vi "EnFlo_Hub.vi"() -> ()   [LabVIEW 2010]
uses:
  Anemometry Sub Vis/Controls/Launch_controls/Open_Calib.ctl
  Anemometry Sub Vis/Controls/Launch_controls/Open_Meas.ctl
  Anemometry Sub Vis/Controls/Launch_controls/Open_Enter_Temp.ctl
  Anemometry Sub Vis/Controls/Launch_controls/Multi_Run_Prog.ctl
  Anemometry Sub Vis/Controls/Launch_controls/EnFlo_arm.ctl
  Anemometry Sub Vis/Controls/Launch_controls/Fast_FID_Valve.ctl
  Anemometry Sub Vis/Controls/Launch_controls/Disp_Setup.ctl
  Anemometry Sub Vis/Controls/Launch_controls/EnFlo_Tun_Setup.ctl
  Anemometry Sub Vis/Controls/Launch_controls/User_Metadata.ctl
  Anemometry Sub Vis/Controls/Launch_controls/Trav_3D_move.ctl
  Anemometry Sub Vis/Controls/Launch_controls/Trav_Space.ctl
  Anemometry Sub Vis/Controls/Launch_controls/Tunnel_speed.ctl
  Anemometry Sub Vis/Controls/Launch_controls/Client_source_control.ctl
  Anemometry Sub Vis/Controls/Launch_controls/Hydrosonic_Manual.ctl
  Anemometry Sub Vis/Controls/Launch_controls/Preference_Panel.ctl
  Anemometry Sub Vis/Controls/Launch_controls/Hot_wire_Calculator.ctl
  Anemometry Sub Vis/Controls/Launch_controls/RW_X_Parker_Config.ctl
  Anemometry Sub Vis/Controls/Launch_controls/LDA_Alignment.ctl
  Anemometry Sub Vis/Controls/Launch_controls/Named_Serial_Comms.ctl
  Anemometry Sub Vis/Controls/Launch_controls/BSA_data_rates.ctl
  Anemometry Sub Vis/Controls/Launch_controls/Recompile_Code.ctl
  Anemometry Sub Vis/Controls/Launch_controls/Serial_Setup.ctl
  Anemometry Sub Vis/Controls/Launch_controls/Post_Process_icon.ctl
  Anemometry Sub Vis/Controls/Launch_controls/Edit_Ascii_file.ctl
  Anemometry Sub Vis/Controls/Launch_controls/Edit_Raw_DF.ctl
  Anemometry Sub Vis/Controls/Launch_controls/Results_file_plotter.ctl
  Anemometry Sub Vis/Controls/Launch_controls/Serial_Port_Names.ctl
  Anemometry Sub Vis/Controls/Launch_controls/Enter_LDA_Setup.ctl
  Anemometry Sub Vis/Controls/Launch_controls/Paul.ctl
  Anemometry Sub Vis/Controls/Launch_controls/Tom.ctl
  Anemometry Sub Vis/Controls/Launch_controls/Scani_Valve.ctl
  Anemometry Sub Vis/Controls/Launch_controls/Edit_sever_Channel.ctl
  Anemometry Sub Vis/Controls/Launch_controls/Day_file_plotter.ctl
  Anemometry Sub Vis/Controls/Launch_controls/Plot_Sever_Data.ctl
  Anemometry Sub Vis/Controls/Launch_controls/Adam_Table.ctl
  Anemometry Sub Vis/Controls/Launch_controls/Active_Channel_Control.ctl
  Anemometry Sub Vis/Controls/Post_Process.ctl
  Anemometry Sub Vis/Controls/Setup.ctl
  Anemometry Sub Vis/Controls/Preference_Mode.ctl
  Anemometry Sub Vis/Controls/User_Specific_mode.ctl
  Anemometry Sub Vis/Gen Trav/Trav_mode.ctl
  Anemometry Sub Vis/File/Setup_Filetype.ctl
  Anemometry Sub Vis/Calibration/Calib_mode.ctl
  Anemometry Sub Vis/Controls/App_Global.ctl
  Anemometry Sub Vis/Globals/Dynamic_call_global.ph.vi
  Anemometry Sub Vis/Globals/Preference_global.vi
  Anemometry Sub Vis/Globals/Constants_global.vi
  Anemometry Sub Vis/Globals/Meas_global.vi
  <vilib>/Platform/browser.llb/Open URL in Default Browser (string).vi
  Anemometry Sub Vis/Globals/Trav_pos_global.vi
  Anemometry Sub Vis/Acquisition/PWA/PWAtasksGLOBAL.vi
  Anemometry Sub Vis/Globals/Qnet_Globals.vi
  Anemometry Sub Vis/Utilities/Email_transfer_global.vi
panel:
  out "List of ADAM channels to view":string[](array[string])
  out "List of ADAM control channels":string[](array[string])
  out "Analogue Dev Name":string="Dev2"
  out "Numeric":i32
  out "Rig Name":string="EnFlo Tunnel"
  out "All Users":path=path "/System Folder/Preferences/LabVIEW (EnFlo specific)/Meas Setups"
  out "Dummy Measurement":bool
  out "Ready to take data?":T1
  out "Local Site Root":path=path "/Lacie_20/paulhayden/Qnet/qnet"
  in  "stop":bool
  in  "Tab Control":T2(tab)
  in  "Tunnel Speed Control":T3
  in  "Traverse Space":T4
  in  "Trav 3D Move":T5 caption="3D Traverse Move"
  in  "User Metadata":T6
  in  "Multi Run Prog":T7
  in  "Enter Temp_Press":T8
  in  "Measurement Prog":T9 caption="Measurement"
  in  "Calibration Prog":T10 caption="Calibration"
  in  "Scani Valve":T11
  in  "LDA Alignment":T12
  in  "Hydrosonic Control":T13
  in  "Fast FID Valve":T14
  in  "Source Control":T15
  in  "Gas Release Setup":T16
  in  "EnFlo Tunnel Setup":T17
  in  "Heater Setup":bool caption="Inlet heater File"
  in  "EnFlo Arm":T18
  in  "Rig_Control":cluster{"Ch Name":string, "Boolean":bool}[](array[cluster])
  in  "ADAM Channels Control":T19 caption="Change Active Channels"
  in  "ADAM Scan Table":T20 caption="Run ADAM Scan Table"
  in  "Edit Server Channel":T21
  in  "Plot Server Channels":T22 caption="Plot Server Data"
  in  "Day Files Plotter":T23 caption="Plot Data From File"
  out "Current Values":cluster{"Ch Name":string, "Numeric":dbl}[](array[cluster])
  in  "Results File Plotter":T24
  in  "Edit Raw Data Files":T25
  in  "Edit ASCII File":T26
  in  "Post Process Raw Data":T27
  in  "LDA Setup":T28
  in  "Port Names":T29
  in  "Serial Setup":T30
  in  "Software Update":T31
  in  "LDA Data Rate":T32
  in  "Named Serial Comms":T33
  in  "RW Trav Setup":T34
  in  "Hot Wire Calc":T35
  in  "Preference Panel":T36
  in  "Tom Lawton t.lawton@surrey.ac.uk":T37 caption="For hardware support"
  in  "Paul Hayden p.hayden@surrey.ac.uk":T38 caption="For software support"
  in  "Online Manual":bool
  out "VI Name":string
  out "Iterations":i32
  # "Or give us a call on Tel: 01483 689545"
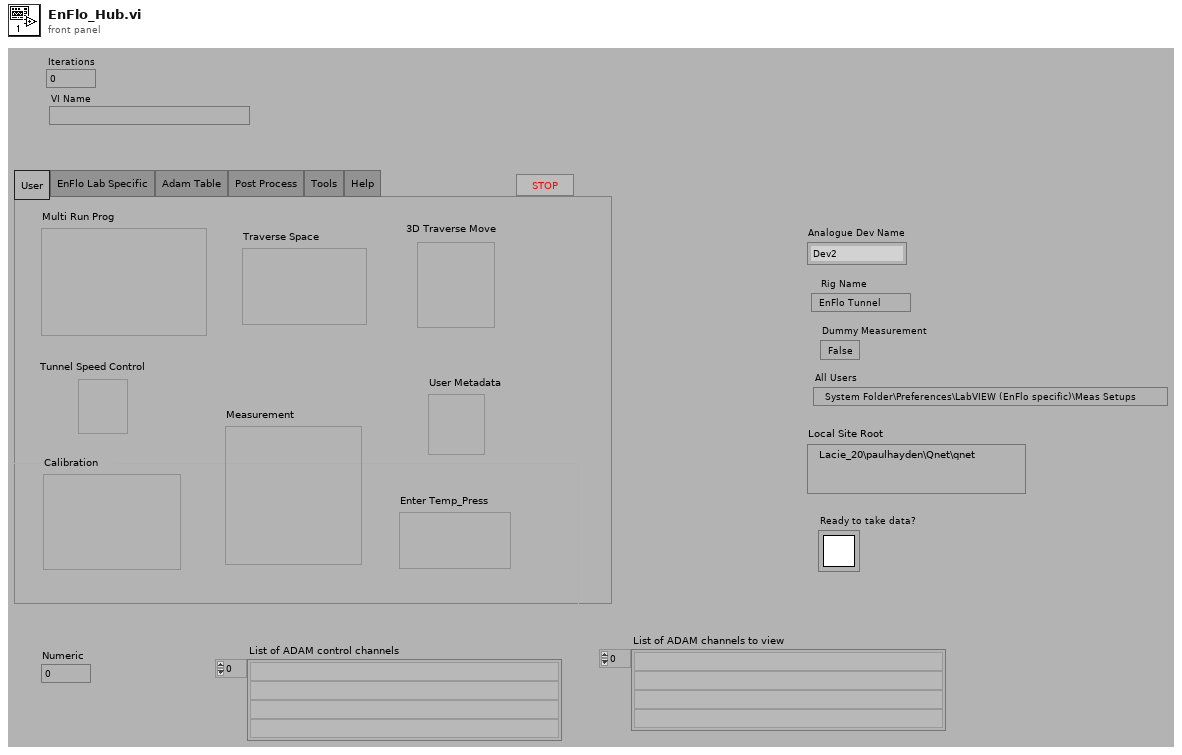
[diagram p1: front panel]
types:
  T1 = typedef "Rendezvous RefNum" = refnum<k1>
  T2 = enum32{"User", "EnFlo Lab Specific", "Adam Table", "Post Process", "Tools", "Help"}
  T3 = typedef "Tunnel_speed.ctl" = bool
  T4 = typedef "Trav_Space.ctl" = bool
  T5 = typedef "Trav_3D_move.ctl" = bool
  T6 = typedef "User_Metadata.ctl" = bool
  T7 = typedef "Multi_Run_Prog.ctl" = bool
  T8 = typedef "Open_Enter_Temp.ctl" = bool
  T9 = typedef "Open_Meas.ctl" = bool
  T10 = typedef "Open_Calib.ctl" = bool
  T11 = typedef "Scani_Valve.ctl" = bool
  T12 = typedef "LDA_Alignment.ctl" = bool
  T13 = typedef "Hydrosonic_Manual.ctl" = bool
  T14 = typedef "Fast_FID_Valve.ctl" = bool
  T15 = typedef "Client_source_control.ctl" = bool
  T16 = typedef "Disp_Setup.ctl" = bool
  T17 = typedef "EnFlo_Tun_Setup.ctl" = bool
  T18 = typedef "EnFlo_arm.ctl" = bool
  T19 = typedef "Active_Channel_Control.ctl" = bool
  T20 = typedef "Adam_Table.ctl" = bool
  T21 = typedef "Edit_sever_Channel.ctl" = bool
  T22 = typedef "Plot_Sever_Data.ctl" = bool
  T23 = typedef "Day_file_plotter.ctl" = bool
  T24 = typedef "Results_file_plotter.ctl" = bool
  T25 = typedef "Edit_Raw_DF.ctl" = bool
  T26 = typedef "Edit_Ascii_file.ctl" = bool
  T27 = typedef "Post_Process_icon.ctl" = bool
  T28 = typedef "Enter_LDA_Setup.ctl" = bool
  T29 = typedef "Serial_Port_Names.ctl" = bool
  T30 = typedef "Serial_Setup.ctl" = bool
  T31 = typedef "Recompile_Code.ctl" = bool
  T32 = typedef "BSA_data_rates.ctl" = bool
  T33 = typedef "Named_Serial_Comms.ctl" = bool
  T34 = typedef "RW_X_Parker_Config.ctl" = bool
  T35 = typedef "Hot_wire_Calculator.ctl" = bool
  T36 = typedef "Preference_Panel.ctl" = bool
  T37 = typedef "Tom.ctl" = bool
  T38 = typedef "Paul.ctl" = bool
  T39 = typedef "Post_Process.ctl" = enum16{"Take New Data", "Post Process Raw Data File"}
  T40 = typedef "Setup.ctl" = enum16{"Run Program", "Show Setup", "Save Current Setup", "Setup Front Panel"}
  T41 = enum16{"Get Channel Names", "Get Current Value", "Update Channel Value", "Update Channel Description"}
  T42 = typedef "Preference_Mode.ctl" = enum16{"Load Preferences from file", "Save Preferences to file", "Load, Edit then Save"}
  T43 = typedef "User_Specific_mode.ctl" = enum16{"Check VI only", "Run VI"}
  T44 = typedef "Trav_mode.ctl" = enum16{"Move traverse", "Read traverse position", "Teach Position"}
  T45 = typedef "Setup_Filetype.ctl" = enum16{"Measurement Setups", "Calibration Setups", "General", "Results File Plotter Setups", "Speed Calib Tweaks"}
  T46 = enum16{"Load Command File", "Save Command File", "Check Multi Run Prog", "Check Multi Run Prog With Live Moves", "Run Multi Run Prog"}
  T47 = typedef "Calib_mode.ctl" = enum16{"Show Setup", "Take a New Calibration Point", "Refit Curve", "Setup Front Panel"}
  T48 = typedef "Tunnel_Coordinates.ctl" = enum16{"Work in Tunnel Coordinates", "Work in Model Coordinates"}
  T49 = typedef "App_Global.ctl" = enum16{"Read Global", "Write to Global", "Initialise Array"}
  T50 = typedef "App_Ref_Cluster.ctl" = cluster{"Server IP & Port No":string, "Application reference":refnum<vi>}
  T51 = typedef "Ch_description_ADAM.ctl" = cluster{"Ch Name":string, "Type":T52, "Function":T53, "Ch State":T54, "Calibration type":T55, "A":dbl, "B":dbl, "C":dbl, "D":dbl, "Comments":string, "Address":T56, "String":string, "Duty":u16}
  T52 = typedef "Module_type_ADAM.ctl" = enum16{"4011", "4012", "4013", "4014", "4016", "4017", "4018", "4021", "4050", "4052", "4053", "4060", "4080", "5000", "5017", "5018", "5024", "5051", "5056", "5060", "6060", "Tracker", "WEST", "GILL", "JEM", "VICI", "Vaisala", "DRUCK", "Run VI Named:", "IR2100", "PPT", "Comparator", "VIRTUAL", "Hold Value", "Read A", "Read Ch", "Coded", "Client Info", "Web Client", "X10", "Test"}
  T53 = typedef "Function_ADAM.ctl" = enum16{"Analogue Input", "Digital Input", "Event counter", "Event rate", "Analogue Output", "Digital Output", "Relay Output"}
  T54 = typedef "Channel_State.ctl" = enum16{"On", "Off", "Always On", "Always Off"}
  T55 = typedef "Calib_type_ADAM.ctl" = enum16{"Raw", "Bx + A", "Cx^2 + Bx + A", "Dx^3 + Cx^2 + Bx + A", "In Band", "Hi-Tec Q", "Hi-Tec M_dot", "Text"}
  T56 = typedef "Address.ctl" = cluster{"Main":i32, "Ch.":i32, "Sub":i32, "Port Name":string}
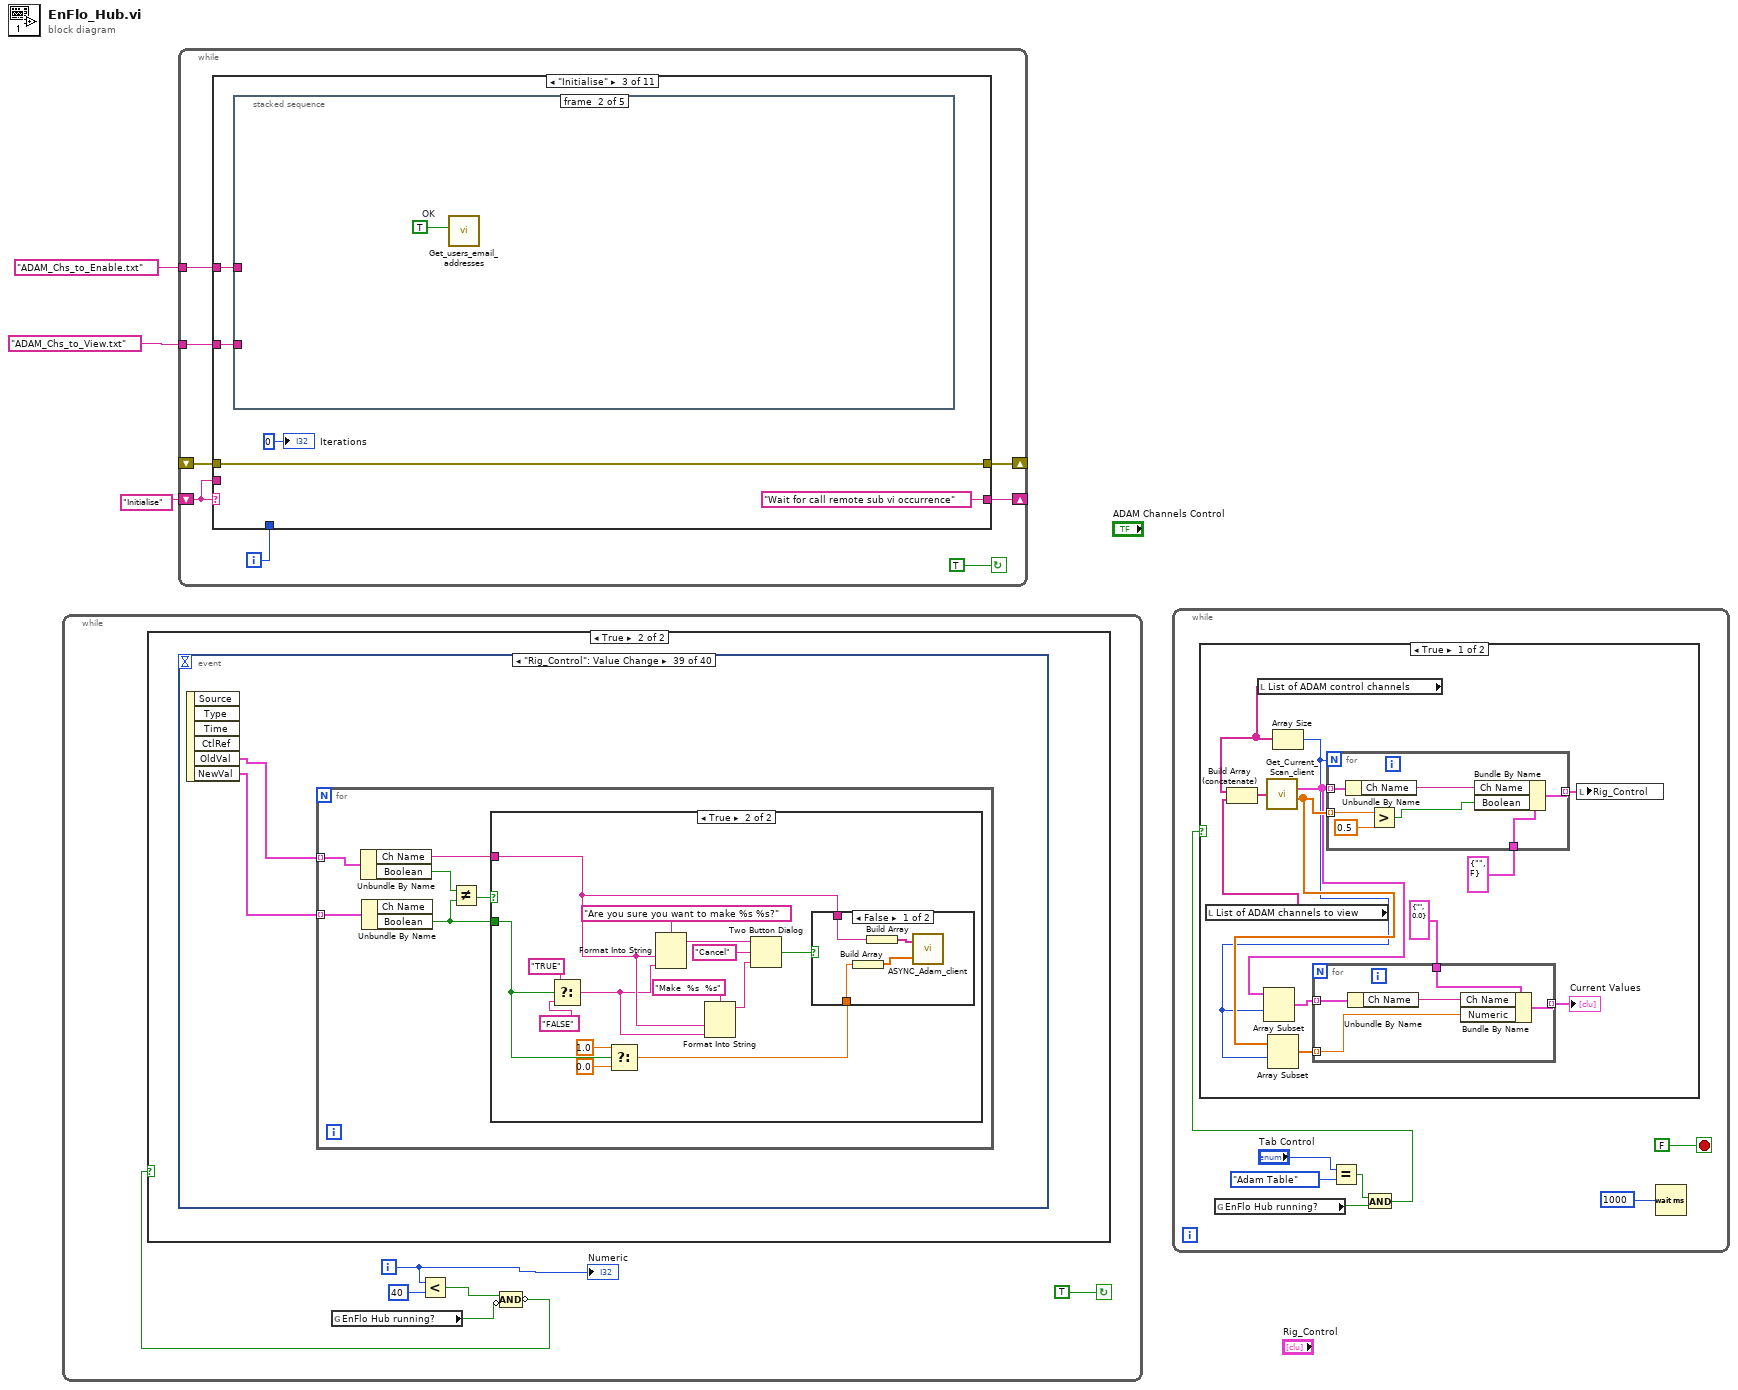
[diagram p0: block diagram]
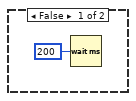
[diagram p3: hidden frame]
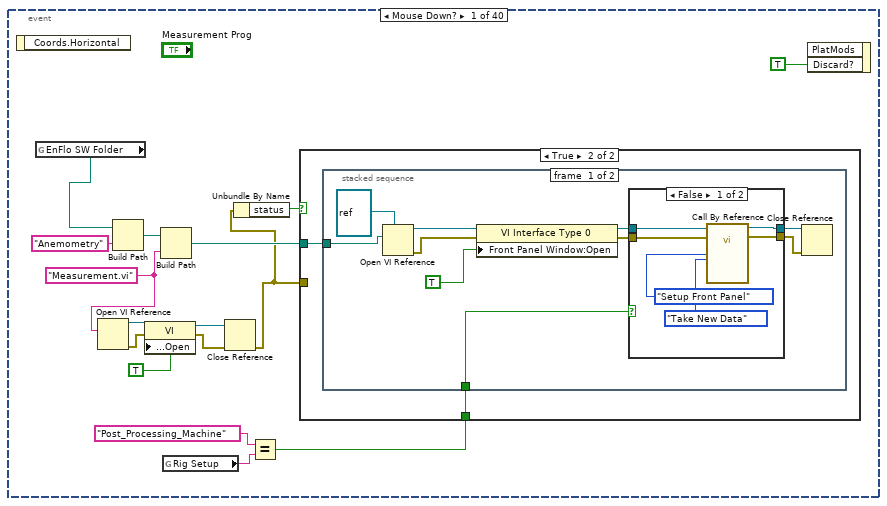
[diagram p4: hidden frame]
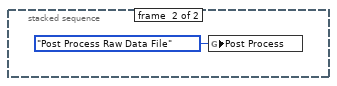
[diagram p7: hidden frame]
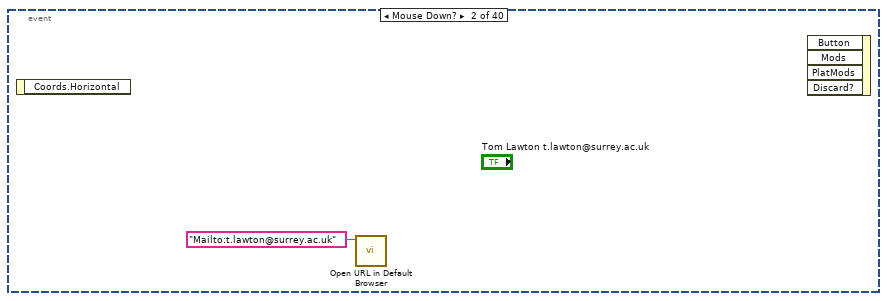
[diagram p8: hidden frame]
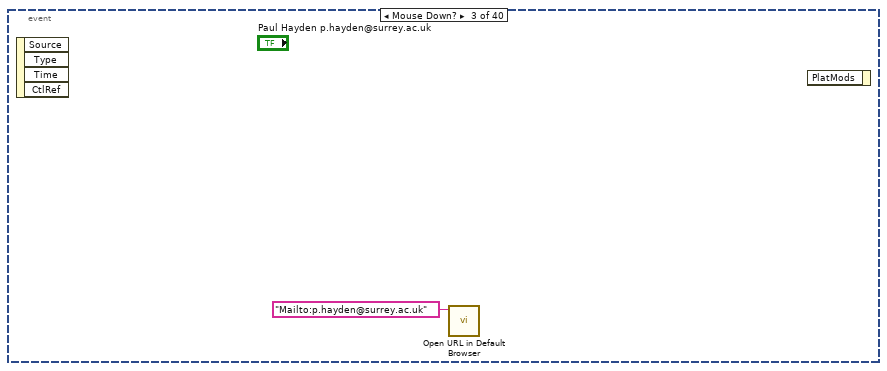
[diagram p9: hidden frame]
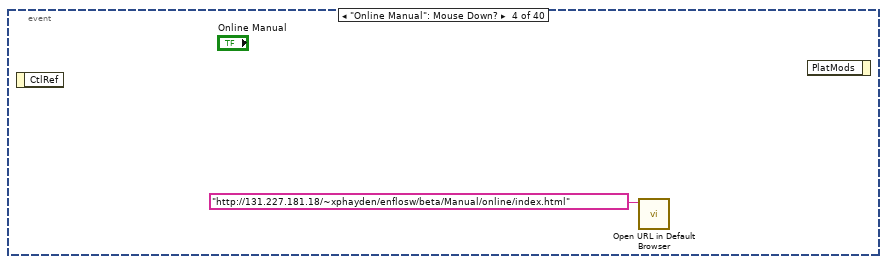
[diagram p10: hidden frame]
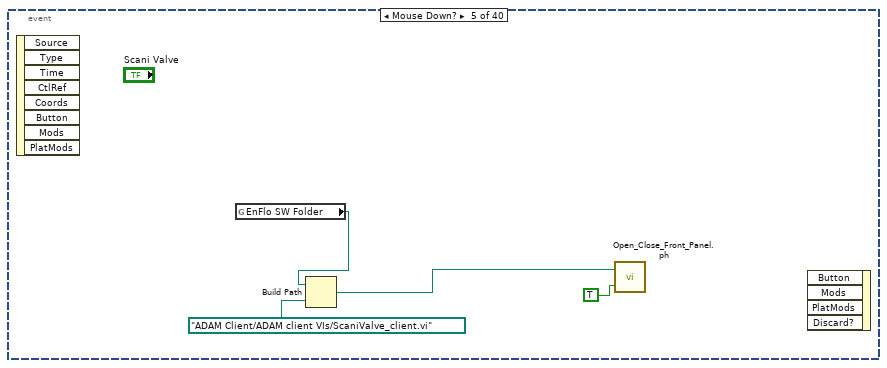
[diagram p11: hidden frame]
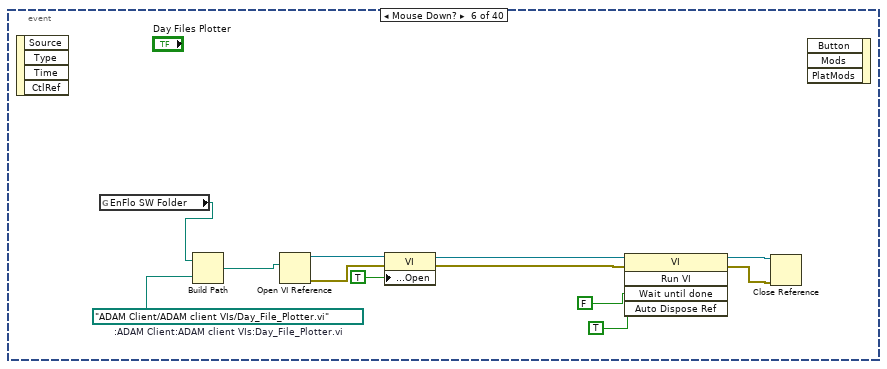
[diagram p12: hidden frame]
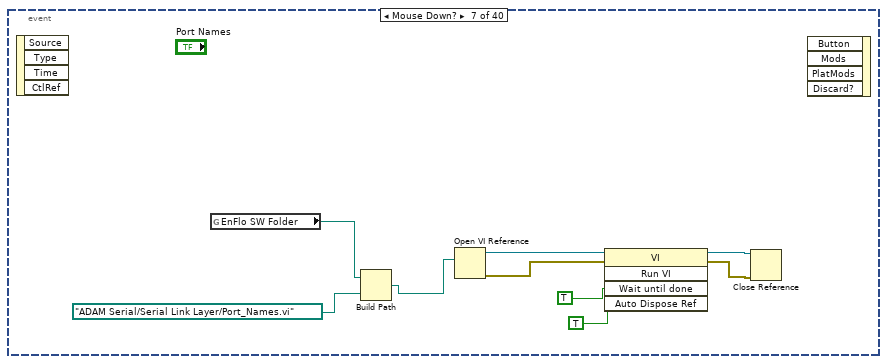
[diagram p13: hidden frame]
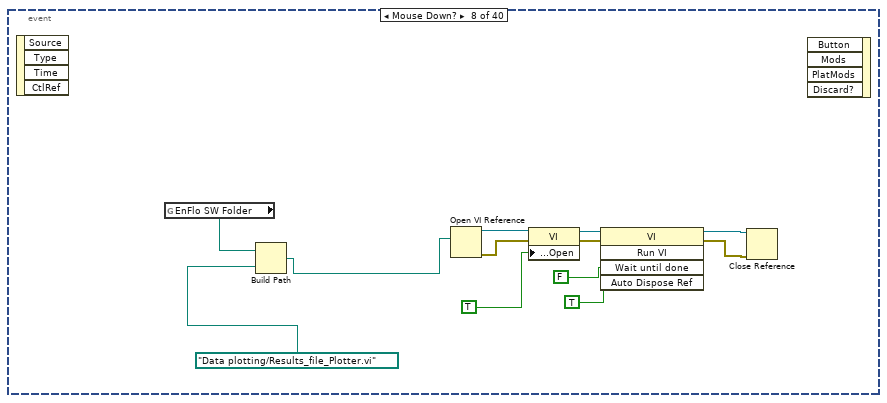
[diagram p14: hidden frame]
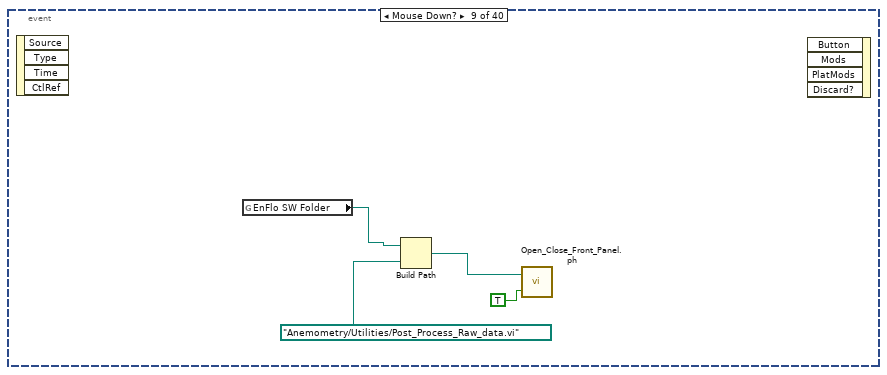
[diagram p15: hidden frame]
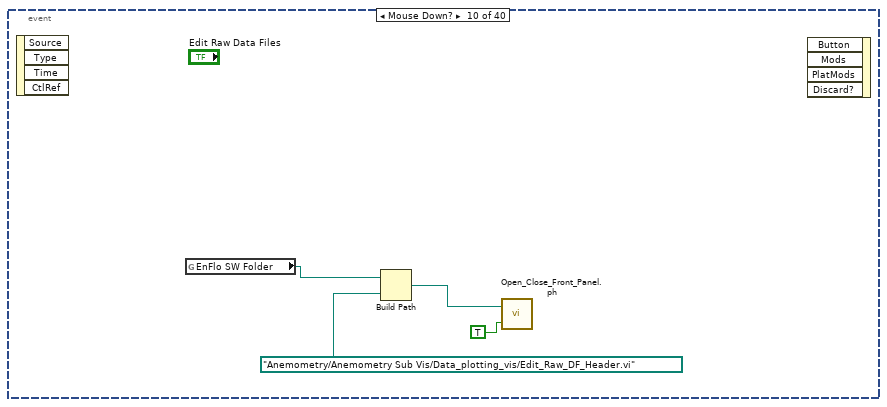
[diagram p16: hidden frame]
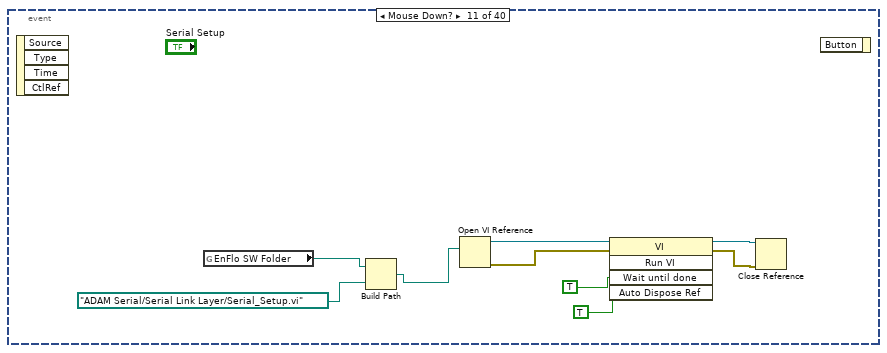
[diagram p17: hidden frame]
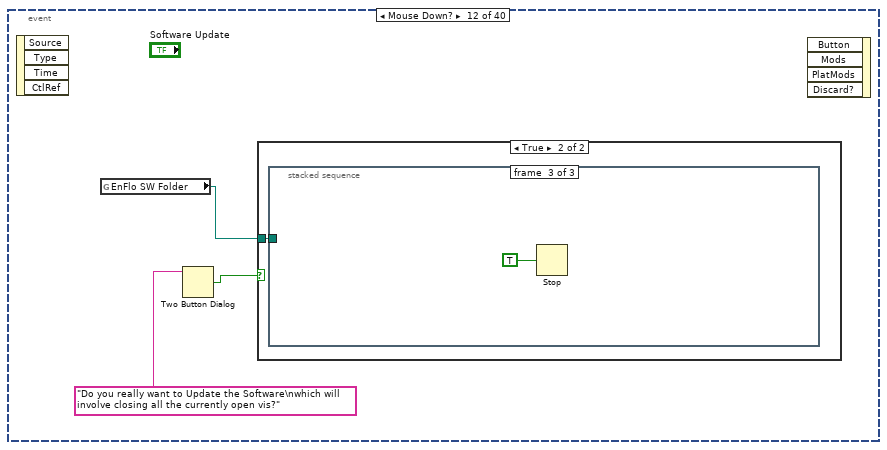
[diagram p18: hidden frame]
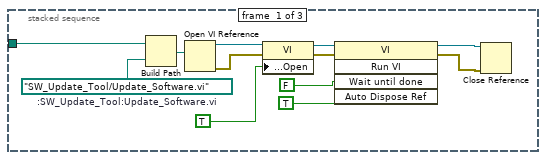
[diagram p20: hidden frame]
diagram:
  n1 = while {
    i -> [w8]
    stop <- TRUE continue-if-true
    n2 = global read "Dynamic_call_global.ph.vi" "EnFlo Hub running?"() -> (w6:bool)
    n3 = Less?(x=w8, y=40) -> (x < y?=w5:bool)
    n4 = Compound Arithmetic op=AND(w5, invert w6) -> (invert w4:bool)
    n5 = case shown="True" w4 {
      frame False {
        n6 = Wait (ms)(milliseconds to wait=u32 200) -> ()  [unwired: 1 out]
      }
      frame True {
        n7 = event shown="[38] \"Rig_Control\": Value Change" {
          selector: _ -> [_ _ _ _ _ _ _ _ _ _ _ _ _ _ _ _ _ _ _ _ _ _ _ _ _ _ _ _ _ _ _ _ _ _ _ _ _ _ _ _]
          dyn-events: _ -> [_ _ _ _ _ _ _ _ _ _ _ _ _ _ _ _ _ _ _ _ _ _ _ _ _ _ _ _ _ _ _ _ _ _ _ _ _ _ _ _]
          timeout: _ -> [_ _ _ _ _ _ _ _ _ _ _ _ _ _ _ _ _ _ _ _ _ _ _ _ _ _ _ _ _ _ _ _ _ _ _ _ _ _ _ _]
          event Mouse Down? {
            w19 = "Measurement.vi" ("name or relative path")
            n8 = event-data() -> ()  [unwired: 2 out]
            n9 = global read "Constants_global.vi" "EnFlo SW Folder"() -> (w22:path)
            n10 = Open VI Reference(vi path=w19) -> (vi reference=w18:refnum<vi>, error out=w17:errorcluster)  [unwired: 1 in, 4 out]
            n11 = Build Path(base path=w22, name or relative path="Anemometry") -> (appended path=w25:path)
            n12 = property class="VI"(reference=w18, error in=w17, "Front Panel Window:Open"=TRUE) -> (reference out=w15:refnum<vi>, error out=w16:errorcluster)
            n13 = Build Path(base path=w25, name or relative path=w19) -> (appended path=w23:path)
            n14 = global read "Preference_global.vi" "Rig Setup"() -> (w13:string)
            n15 = Close Reference(reference=w15, error in (no error)=w16) -> (error out=w14:errorcluster)
            n16 = Unbundle By Name(w14) -> ("status"=w24:bool)
            n17 = Equal?(x="Post_Processing_Machine" ("Rig Setup"), y=w13) -> (x = y?=w11:bool)
            n18 = case shown="True" w24 {
              tunnel: w23 -> [_ w28]
              tunnel: w14 -> [_ _]
              tunnel: w11 -> [_ w27]
              frame False {
              }
              frame True {
                n19 = stacked-sequence {
                  tunnel: w28 -> [w38 _]
                  tunnel: w27 -> [w29 _]
                  frame #0 {
                    n20 = Open VI Reference(type specifier VI Refnum (for type only)=refnum<vi> refnum, vi path=w38) -> (vi reference=w36:refnum<vi>, error out=w35:errorcluster)  [unwired: 1 in, 3 out]
                    n21 = property class="VI Interface Type 0"(reference=w36, error in=w35, "Front Panel Window:Open"=TRUE) -> (reference out=w31:refnum<vi>, error out=w30:errorcluster)
                    n22 = case shown="False" w29 {
                      tunnel: [w44 w46] -> w34
                      tunnel: [w43 w45] -> w33
                      tunnel: w31 -> [w42 w46]
                      tunnel: w30 -> [w41 w45]
                      frame False {
                        n23 = call-by-ref "?"(reference=w42, error in=w41, "setup"=Setup."Setup Front Panel", "Post Process"=Post_Process."Take New Data") -> (reference out=w44:refnum<vi>, error out=w43:errorcluster)  [unwired: 16 in, 2 out]
                      }
                      frame True {
                      }
                    }
                    n24 = Close Reference(reference=w34, error in (no error)=w33) -> ()  [unwired: 1 out]
                  }
                  frame #1 {
                    n25 = global write "Meas_global.vi" "Post Process"(Post_Process."Post Process Raw Data File" ("Post Process")) -> ()
                  }
                }
              }
            }
            n26 = event-data("Discard?"=TRUE) -> ()  [unwired: 1 in, 2 out]
          }
          event Mouse Down? {
            n27 = event-data() -> ()  [unwired: 2 out]
            n28 = call-poly <vilib>:"Open URL in Default Browser.vi"("URL"="Mailto:t.lawton@surrey.ac.uk") -> ()  [unwired: 1 in, 6 out]
            n29 = event-data() -> ()  [unwired: 1 in, 5 out]
          }
          event Mouse Down? {
            n30 = event-data() -> ()  [unwired: 5 out]
            n31 = call-poly <vilib>:"Open URL in Default Browser.vi"("URL"="Mailto:p.hayden@surrey.ac.uk") -> ()  [unwired: 1 in, 6 out]
            n32 = event-data() -> ()  [unwired: 1 in, 2 out]
          }
          event "Online Manual": Mouse Down? {
            n33 = event-data() -> ()  [unwired: 2 out]
            n34 = call-poly <vilib>:"Open URL in Default Browser.vi"("URL"="http://131.227.181.18/~xphayden/enflosw/beta/Manual/online/index.html") -> ()  [unwired: 1 in, 6 out]
            n35 = event-data() -> ()  [unwired: 1 in, 2 out]
          }
          event Mouse Down? {
            n36 = event-data() -> ()  [unwired: 9 out]
            n37 = global read "Constants_global.vi" "EnFlo SW Folder"() -> (w51:path)
            n38 = Build Path(base path=w51, name or relative path=path "ADAM Client/ADAM client VIs/ScaniValve_client.vi") -> (appended path=w54:path)
            n39 = call "Open_Close_Front_Panel.ph.vi"("Front Panel Window:Open"=TRUE, "VI path"=w54) -> ()  [unwired: 2 out]
            n40 = event-data() -> ()  [unwired: 1 in, 5 out]
          }
          event Mouse Down? {
            w56 = path "ADAM Client/ADAM client VIs/Day_File_Plotter.vi"  # :ADAM Client:ADAM client VIs:Day_File_Plotter.vi
            n41 = event-data() -> ()  [unwired: 5 out]
            n42 = global read "Constants_global.vi" "EnFlo SW Folder"() -> (w55:path)
            n43 = Build Path(base path=w55, name or relative path=w56) -> (appended path=w61:path)
            n44 = Open VI Reference(vi path=w61) -> (vi reference=w62:refnum<vi>, error out=w64:errorcluster)  [unwired: 2 in, 3 out]
            n45 = property class="VI"(reference=w62, error in=w64, "Front Panel Window:Open"=TRUE) -> (reference out=w66:refnum<vi>, error out=w65:errorcluster)
            n46 = invoke class="VI" method="Run VI"(reference=w66, error in=w65, "Wait until done"=FALSE, "Auto Dispose Ref"=TRUE) -> (reference out=w57:refnum<vi>, error out=w58:errorcluster)  [unwired: 1 in, 3 out]
            n47 = Close Reference(reference=w57, error in (no error)=w58) -> ()  [unwired: 1 out]
            n48 = event-data() -> ()  [unwired: 1 in, 4 out]
          }
          event Mouse Down? {
            n49 = event-data() -> ()  [unwired: 5 out]
            n50 = global read "Constants_global.vi" "EnFlo SW Folder"() -> (w67:path)
            n51 = Build Path(base path=w67, name or relative path=path "ADAM Serial/Serial Link Layer/Port_Names.vi") -> (appended path=w69:path)
            n52 = Open VI Reference(vi path=w69) -> (vi reference=w74:refnum<vi>, error out=w75:errorcluster)  [unwired: 1 in, 4 out]
            n53 = invoke class="VI" method="Run VI"(reference=w74, error in=w75, "Wait until done"=TRUE, "Auto Dispose Ref"=TRUE) -> (reference out=w70:refnum<vi>, error out=w71:errorcluster)  [unwired: 1 in, 3 out]
            n54 = Close Reference(reference=w70, error in (no error)=w71) -> ()  [unwired: 1 out]
            n55 = event-data() -> ()  [unwired: 1 in, 5 out]
          }
          event Mouse Down? {
            n56 = event-data() -> ()  [unwired: 5 out]
            n57 = global read "Constants_global.vi" "EnFlo SW Folder"() -> (w76:path)
            n58 = Build Path(base path=w76, name or relative path=path "Data plotting/Results_file_Plotter.vi") -> (appended path=w79:path)
            n59 = Open VI Reference(vi path=w79) -> (vi reference=w81:refnum<vi>, error out=w78:errorcluster)  [unwired: 1 in, 4 out]
            n60 = property class="VI"(reference=w81, error in=w78, "Front Panel Window:Open"=TRUE) -> (reference out=w82:refnum<vi>, error out=w83:errorcluster)
            n61 = invoke class="VI" method="Run VI"(reference=w82, error in=w83, "Wait until done"=FALSE, "Auto Dispose Ref"=TRUE) -> (reference out=w84:refnum<vi>, error out=w85:errorcluster)  [unwired: 1 in, 3 out]
            n62 = Close Reference(reference=w84, error in (no error)=w85) -> ()  [unwired: 1 out]
            n63 = event-data() -> ()  [unwired: 1 in, 5 out]
          }
          event Mouse Down? {
            n64 = event-data() -> ()  [unwired: 5 out]
            n65 = global read "Constants_global.vi" "EnFlo SW Folder"() -> (w88:path)
            n66 = Build Path(base path=w88, name or relative path=path "Anemometry/Utilities/Post_Process_Raw_data.vi") -> (appended path=w90:path)
            n67 = call "Open_Close_Front_Panel.ph.vi"("Front Panel Window:Open"=TRUE, "VI path"=w90) -> ()  [unwired: 2 out]
            n68 = event-data() -> ()  [unwired: 1 in, 5 out]
          }
          event Mouse Down? {
            n69 = event-data() -> ()  [unwired: 5 out]
            n70 = global read "Constants_global.vi" "EnFlo SW Folder"() -> (w92:path)
            n71 = Build Path(base path=w92, name or relative path=path "Anemometry/Anemometry Sub Vis/Data_plotting_vis/Edit_Raw_DF_Header.vi") -> (appended path=w94:path)
            n72 = call "Open_Close_Front_Panel.ph.vi"("Front Panel Window:Open"=TRUE, "VI path"=w94) -> ()  [unwired: 2 out]
            n73 = event-data() -> ()  [unwired: 1 in, 5 out]
          }
          event Mouse Down? {
            n74 = event-data() -> ()  [unwired: 5 out]
            n75 = global read "Constants_global.vi" "EnFlo SW Folder"() -> (w96:path)
            n76 = Build Path(base path=w96, name or relative path=path "ADAM Serial/Serial Link Layer/Serial_Setup.vi") -> (appended path=w98:path)
            n77 = Open VI Reference(vi path=w98) -> (vi reference=w103:refnum<vi>, error out=w104:errorcluster)  [unwired: 1 in, 4 out]
            n78 = invoke class="VI" method="Run VI"(reference=w103, error in=w104, "Wait until done"=TRUE, "Auto Dispose Ref"=TRUE) -> (reference out=w99:refnum<vi>, error out=w100:errorcluster)  [unwired: 1 in, 3 out]
            n79 = Close Reference(reference=w99, error in (no error)=w100) -> ()  [unwired: 1 out]
            n80 = event-data() -> ()  [unwired: 1 in, 2 out]
          }
          event Mouse Down? {
            n81 = event-data() -> ()  [unwired: 5 out]
            n82 = global read "Constants_global.vi" "EnFlo SW Folder"() -> (w105:path)
            n83 = Two Button Dialog(message="Do you really want to Update the Software\nwhich will involve closing all the currently open vis?") -> (T button?=w107:bool)  [unwired: 2 out]
            n84 = case shown="True" w107 {
              tunnel: w105 -> [_ w108]
              frame False {
              }
              frame True {
                n85 = stacked-sequence {
                  tunnel: w108 -> [w120 _ _]
                  frame #0 {
                    w109 = path "SW_Update_Tool/Update_Software.vi"  # :SW_Update_Tool:Update_Software.vi
                    n86 = Build Path(base path=w120, name or relative path=w109) -> (appended path=w118:path)
                    n87 = Open VI Reference(vi path=w118) -> (vi reference=w116:refnum<vi>, error out=w119:errorcluster)  [unwired: 1 in, 4 out]
                    n88 = property class="VI"(reference=w116, error in=w119, "Front Panel Window:Open"=TRUE) -> (reference out=w115:refnum<vi>, error out=w114:errorcluster)
                    n89 = invoke class="VI" method="Run VI"(reference=w115, error in=w114, "Wait until done"=FALSE, "Auto Dispose Ref"=TRUE) -> (reference out=w113:refnum<vi>, error out=w112:errorcluster)  [unwired: 1 in, 3 out]
                    n90 = Close Reference(reference=w113, error in (no error)=w112) -> ()  [unwired: 1 out]
                  }
                  frame #1 {
                    n91 = global write "Dynamic_call_global.ph.vi" "EnFlo Hub running?"(FALSE ("EnFlo Hub running?")) -> ()
                  }
                  frame #2 {
                    n92 = Stop(stop? (T)=TRUE) -> ()
                  }
                }
              }
            }
            n93 = event-data() -> ()  [unwired: 1 in, 5 out]
          }
          event Mouse Down? {
            n94 = event-data() -> ()  [unwired: 5 out]
            n95 = global read "Constants_global.vi" "EnFlo SW Folder"() -> (w124:path)
            n96 = Build Path(base path=w124, name or relative path=path "ADAM Serial/Serial Link Layer/Named_Serial_Comms.vi") -> (appended path=w126:path)
            n97 = call "Open_Close_Front_Panel.ph.vi"("Front Panel Window:Open"=TRUE, "VI path"=w126) -> ()  [unwired: 2 out]
            n98 = event-data() -> ()  [unwired: 1 in, 5 out]
          }
          event Mouse Down? {
            n99 = event-data() -> ()  [unwired: 5 out]
            n100 = global read "Constants_global.vi" "EnFlo SW Folder"() -> (w127:path)
            n101 = Build Path(base path=w127, name or relative path=path "Anemometry/Anemometry Sub Vis/LDA/LDA_data_rate.vi") -> (appended path=w129:path)
            n102 = call "Open_Close_Front_Panel.ph.vi"("Front Panel Window:Open"=TRUE, "VI path"=w129) -> ()  [unwired: 2 out]
            n103 = event-data() -> ()  [unwired: 1 in, 2 out]
          }
          event Mouse Down? {
            n104 = event-data() -> ()  [unwired: 5 out]
            n105 = global read "Constants_global.vi" "EnFlo SW Folder"() -> (w141:path)
            n106 = Build Path(base path=w141, name or relative path=path "ADAM Client/ADAM client VIs/Control_Channel_Status.vi") -> (appended path=w131:path)
            n107 = Open VI Reference(vi path=w131) -> (vi reference=w134:refnum<vi>, error out=w132:errorcluster)  [unwired: 1 in, 4 out]
            n108 = property class="VI"(reference=w134, error in=w132, "Front Panel Window:Open"=TRUE) -> (reference out=w135:refnum<vi>, error out=w136:errorcluster)
            n109 = invoke class="VI" method="Run VI"(reference=w135, error in=w136, "Wait until done"=FALSE, "Auto Dispose Ref"=TRUE) -> (reference out=w137:refnum<vi>, error out=w138:errorcluster)  [unwired: 1 in, 3 out]
            n110 = Close Reference(reference=w137, error in (no error)=w138) -> ()  [unwired: 1 out]
            n111 = event-data() -> ()  [unwired: 1 in, 2 out]
          }
          event Mouse Down? {
            n112 = event-data() -> ()  [unwired: 5 out]
            n113 = global read "Constants_global.vi" "EnFlo SW Folder"() -> (w143:path)
            n114 = Build Path(base path=w143, name or relative path=path "Anemometry/Utilities/LDA_Beam_Alignment.vi") -> (appended path=w145:path)
            n115 = call "Open_Close_Front_Panel.ph.vi"("Front Panel Window:Open"=TRUE, "VI path"=w145) -> ()  [unwired: 2 out]
            n116 = event-data() -> ()  [unwired: 1 in, 5 out]
          }
          event Mouse Down? {
            w148 = FALSE  # Wait until done
            n117 = event-data() -> ()  [unwired: 5 out]
            n118 = call "Run_Enter_Temp.vi"("Wait until done"=w148) -> ()  [unwired: 1 out]
            n119 = event-data("Discard?"=TRUE) -> ()  [unwired: 1 in, 4 out]
          }
          event Mouse Down? {
            n120 = event-data() -> ()  [unwired: 5 out]
            n121 = global read "Constants_global.vi" "EnFlo SW Folder"() -> (w149:path)
            n122 = Build Path(base path=w149, name or relative path=path "Anemometry/Utilities/Edit_ASCI_file.vi") -> (appended path=w152:path)
            n123 = call "Open_Close_Front_Panel.ph.vi"("Front Panel Window:Open"=TRUE, "VI path"=w152) -> ()  [unwired: 2 out]
            n124 = event-data() -> ()  [unwired: 1 in, 5 out]
          }
          event "Heater Setup": Mouse Down? {
            w155 = path "Anemometry/Utilities/Create_Heater_Setpoints_File.vi"  # :Anemometry:Utilities:Create_Heater_Setpoints_File.vi
            n125 = event-data() -> ()  [unwired: 5 out]
            n126 = global read "Constants_global.vi" "EnFlo SW Folder"() -> (w153:path)
            n127 = Build Path(base path=w153, name or relative path=w155) -> (appended path=w156:path)
            n128 = call "Open_Close_Front_Panel.ph.vi"("Front Panel Window:Open"=TRUE, "VI path"=w156) -> ()  [unwired: 2 out]
            n129 = event-data() -> ()  [unwired: 1 in, 5 out]
          }
          event Mouse Down? {
            n130 = event-data() -> ()  [unwired: 5 out]
            n131 = global read "Constants_global.vi" "EnFlo SW Folder"() -> (w157:path)
            n132 = Build Path(base path=w157, name or relative path=path "ADAM Client/Sub VIs/Gas_Release_Control.vi") -> (appended path=w160:path)
            n133 = call "Open_Close_Front_Panel.ph.vi"("Front Panel Window:Open"=TRUE, "VI path"=w160) -> ()  [unwired: 2 out]
            n134 = event-data() -> ()  [unwired: 1 in, 5 out]
          }
          event Mouse Down? {
            n135 = event-data() -> ()  [unwired: 5 out]
            n136 = global read "Constants_global.vi" "EnFlo SW Folder"() -> (w161:path)
            n137 = Build Path(base path=w161, name or relative path=path "ADAM Client/ADAM client VIs/Edit_Server_Channel.vi") -> (appended path=w171:path)
            n138 = Open VI Reference(type specifier VI Refnum (for type only)=refnum<vi> refnum, vi path=w171) -> (vi reference=w164:refnum<vi>, error out=w165:errorcluster)  [unwired: 1 in, 3 out]
            n139 = property class="VI Interface Type 1"(reference=w164, error in=w165, "Front Panel Window:Open"=TRUE) -> (reference out=w167:refnum<vi>, error out=w168:errorcluster)
            n140 = call-by-ref "?"(reference=w167, error in=w168, "Mode"=T41."Get Channel Names") -> (reference out=w169:refnum<vi>, error out=w170:errorcluster)  [unwired: 5 in]
            n141 = Close Reference(reference=w169, error in (no error)=w170) -> ()  [unwired: 1 out]
            n142 = event-data() -> ()  [unwired: 1 in, 5 out]
          }
          event Mouse Down? {
            n143 = event-data() -> ()  [unwired: 5 out]
            n144 = global read "Constants_global.vi" "EnFlo SW Folder"() -> (w173:path)
            n145 = Build Path(base path=w173, name or relative path=path "ADAM Client/ADAM client VIs/Set_Tunnel_Speed.vi") -> (appended path=w176:path)
            n146 = call "Open_Close_Front_Panel.ph.vi"("Front Panel Window:Open"=TRUE, "VI path"=w176) -> ()  [unwired: 2 out]
            n147 = event-data() -> ()  [unwired: 1 in, 5 out]
          }
          event Mouse Down? {
            n148 = event-data() -> ()  [unwired: 5 out]
            n149 = global read "Constants_global.vi" "EnFlo SW Folder"() -> (w177:path)
            n150 = Build Path(base path=w177, name or relative path=path "ADAM Client/ADAM client VIs/Plot_Server_Data.vi") -> (appended path=w180:path)
            n151 = Open VI Reference(vi path=w180) -> (vi reference=w182:refnum<vi>, error out=w179:errorcluster)  [unwired: 1 in, 4 out]
            n152 = property class="VI"(reference=w182, error in=w179, "Front Panel Window:Open"=TRUE) -> (reference out=w183:refnum<vi>, error out=w184:errorcluster)
            n153 = invoke class="VI" method="Run VI"(reference=w183, error in=w184, "Wait until done"=FALSE, "Auto Dispose Ref"=TRUE) -> (reference out=w185:refnum<vi>, error out=w186:errorcluster)  [unwired: 1 in, 3 out]
            n154 = Close Reference(reference=w185, error in (no error)=w186) -> ()  [unwired: 1 out]
            n155 = event-data() -> ()  [unwired: 1 in, 5 out]
          }
          event Mouse Down? {
            n156 = event-data() -> ()  [unwired: 5 out]
            n157 = Two Button Dialog(message="Are you sure that you want to Run the ADAM Scan table on this machine?", 1:"Run" ("F button name (\"Cancel\")"), 2:"Cancel" ("T button name (\"OK\")")) -> (T button?=w190:bool)
            n158 = case shown="False" w190 {
              frame False {
                w194 = path "ADAM Server/ADAM_scan_table.vi"  # :ADAM Server:ADAM_scan_table.vi
                n159 = global read "Constants_global.vi" "EnFlo SW Folder"() -> (w193:path)
                n160 = Build Path(base path=w193, name or relative path=w194) -> (appended path=w196:path)
                n161 = Open VI Reference(vi path=w196) -> (vi reference=w198:refnum<vi>, error out=w195:errorcluster)  [unwired: 1 in, 4 out]
                n162 = property class="VI"(reference=w198, error in=w195, "Front Panel Window:Open"=TRUE) -> (reference out=w199:refnum<vi>, error out=w200:errorcluster)
                n163 = invoke class="VI" method="Run VI"(reference=w199, error in=w200, "Wait until done"=FALSE, "Auto Dispose Ref"=TRUE) -> (reference out=w201:refnum<vi>, error out=w202:errorcluster)  [unwired: 1 in, 3 out]
                n164 = Close Reference(reference=w201, error in (no error)=w202) -> ()  [unwired: 1 out]
              }
              frame True {
              }
            }
            n165 = event-data() -> ()  [unwired: 1 in, 2 out]
          }
          event Mouse Down? {
            n166 = event-data() -> ()  [unwired: 5 out]
            n167 = global read "Constants_global.vi" "EnFlo SW Folder"() -> (w207:path)
            n168 = Build Path(base path=w207, name or relative path=path "ADAM Serial/Instrument drivers/Traverses/~subVIs/Read_Write_Trav_Config.vi") -> (appended path=w208:path)
            n169 = Build Path(base path=w207, name or relative path=path "ADAM Serial/Instrument drivers/Traverses/~subVIs/DriveConfigGlobal.vi") -> (appended path=w209:path)
            n170 = flat-sequence {
              tunnel: w209 -> [w210]
              tunnel: w208 -> [w212]
              frame #0 {
                n171 = call "Open_Close_Front_Panel.ph.vi"("Front Panel Window:Open"=TRUE, "VI path"=w210) -> ()  [unwired: 2 out]
              }
              frame #1 {
                n172 = call "Open_Close_Front_Panel.ph.vi"("Front Panel Window:Open"=TRUE, "VI path"=w212) -> ()  [unwired: 2 out]
              }
            }
            n173 = event-data() -> ()  [unwired: 1 in, 5 out]
          }
          event Mouse Down? {
            n174 = event-data() -> ()  [unwired: 5 out]
            n175 = global read "Constants_global.vi" "EnFlo SW Folder"() -> (w214:path)
            n176 = Build Path(base path=w214, name or relative path=path "Anemometry/Utilities/Hot_wire_Calculator.vi") -> (appended path=w217:path)
            n177 = call "Open_Close_Front_Panel.ph.vi"("Front Panel Window:Open"=TRUE, "VI path"=w217) -> ()  [unwired: 2 out]
            n178 = event-data() -> ()  [unwired: 1 in, 5 out]
          }
          event Mouse Down? {
            n179 = event-data() -> ()  [unwired: 5 out]
            n180 = global read "Constants_global.vi" "EnFlo SW Folder"() -> (w218:path)
            n181 = Build Path(base path=w218, name or relative path=path "Anemometry/Utilities/Hydrosonic_Manual.vi") -> (appended path=w221:path)
            n182 = call "Open_Close_Front_Panel.ph.vi"("Front Panel Window:Open"=TRUE, "VI path"=w221) -> ()  [unwired: 2 out]
            n183 = event-data() -> ()  [unwired: 1 in, 5 out]
          }
          event Mouse Down? {
            n184 = event-data() -> ()  [unwired: 5 out]
            n185 = global read "Constants_global.vi" "EnFlo SW Folder"() -> (w222:path)
            n186 = Build Path(base path=w222, name or relative path=path "ADAM Client/ADAM client VIs/Fast_FID_Valve_Control.vi") -> (appended path=w225:path)
            n187 = call "Open_Close_Front_Panel.ph.vi"("Front Panel Window:Open"=TRUE, "VI path"=w225) -> ()  [unwired: 2 out]
            n188 = event-data() -> ()  [unwired: 1 in, 5 out]
          }
          event Mouse Down? {
            n189 = event-data() -> ()  [unwired: 5 out]
            n190 = global read "Constants_global.vi" "EnFlo SW Folder"() -> (w226:path)
            n191 = Build Path(base path=w226, name or relative path=path "Anemometry/Utilities/Preference_Panel.vi") -> (appended path=w235:path)
            n192 = Open VI Reference(type specifier VI Refnum (for type only)=refnum<vi> refnum, vi path=w235) -> (vi reference=w228:refnum<vi>, error out=w229:errorcluster)  [unwired: 1 in, 3 out]
            n193 = property class="VI Interface Type 2"(reference=w228, error in=w229, "Front Panel Window:Open"=TRUE) -> (reference out=w231:refnum<vi>, error out=w232:errorcluster)
            n194 = call-by-ref "?"(reference=w231, error in=w232, "Mode"=Preference_Mode."Load, Edit then Save") -> (reference out=w233:refnum<vi>, error out=w234:errorcluster)
            n195 = Close Reference(reference=w233, error in (no error)=w234) -> ()  [unwired: 1 out]
            n196 = event-data("Discard?"=TRUE) -> ()  [unwired: 1 in, 4 out]
          }
          event Mouse Down? {
            n197 = event-data() -> ()  [unwired: 5 out]
            n198 = global read "Constants_global.vi" "EnFlo SW Folder"() -> (w242:path)
            n199 = Build Path(base path=w242, name or relative path=path "ADAM Client/Sub VIs/Gas_Setup.vi") -> (appended path=w249:path)
            n200 = Open VI Reference(type specifier VI Refnum (for type only)=refnum<vi> refnum, vi path=w249) -> (vi reference=w245:refnum<vi>, error out=w246:errorcluster)  [unwired: 1 in, 3 out]
            n201 = property class="VI Interface Type 3"(reference=w245, error in=w246, "Front Panel Window:Open"=TRUE) -> (reference out=w250:refnum<vi>, error out=w248:errorcluster)
            n202 = call-by-ref "?"(reference=w250, error in=w248) -> (reference out=w240:refnum<vi>, error out=w239:errorcluster)  [unwired: 9 in]
            n203 = Close Reference(reference=w240, error in (no error)=w239) -> ()  [unwired: 1 out]
            n204 = event-data("Discard?"=TRUE) -> ()  [unwired: 1 in, 4 out]
          }
          event Mouse Down? {
            n205 = event-data() -> ()  [unwired: 5 out]
            n206 = global read "Constants_global.vi" "EnFlo SW Folder"() -> (w254:path)
            n207 = Build Path(base path=w254, name or relative path=path "ADAM Client/Sub VIs/User_Metadata.vi") -> (appended path=w261:path)
            n208 = Open VI Reference(type specifier VI Refnum (for type only)=refnum<vi> refnum, vi path=w261) -> (vi reference=w257:refnum<vi>, error out=w258:errorcluster)  [unwired: 1 in, 3 out]
            n209 = property class="VI Interface Type 3"(reference=w257, error in=w258, "Front Panel Window:Open"=TRUE) -> (reference out=w262:refnum<vi>, error out=w260:errorcluster)
            n210 = call-by-ref "?"(reference=w262, error in=w260) -> (reference out=w252:refnum<vi>, error out=w251:errorcluster)  [unwired: 9 in]
            n211 = Close Reference(reference=w252, error in (no error)=w251) -> ()  [unwired: 1 out]
            n212 = event-data("Discard?"=TRUE) -> ()  [unwired: 1 in, 4 out]
          }
          event Mouse Down? {
            n213 = event-data() -> ()  [unwired: 5 out]
            n214 = global read "Constants_global.vi" "EnFlo SW Folder"() -> (w268:path)
            n215 = Build Path(base path=w268, name or relative path=path "ADAM Client/Sub VIs/EnFlo_Tunnel_Setup.vi") -> (appended path=w271:path)
            n216 = Open VI Reference(type specifier VI Refnum (for type only)=refnum<vi> refnum, vi path=w271) -> (vi reference=w265:refnum<vi>, error out=w264:errorcluster)  [unwired: 1 in, 3 out]
            n217 = call-by-ref "?"(reference=w265, error in=w264) -> (reference out=w267:refnum<vi>, error out=w266:errorcluster)  [unwired: 9 in]
            n218 = Close Reference(reference=w267, error in (no error)=w266) -> ()  [unwired: 1 out]
            n219 = event-data("Discard?"=TRUE) -> ()  [unwired: 1 in, 4 out]
          }
          event Mouse Down? {
            w282 = TRUE  # Show Panel?
            n220 = event-data() -> ()  [unwired: 5 out]
            n221 = global read "Constants_global.vi" "EnFlo SW Folder"() -> (w277:path)
            n222 = Build Path(base path=w277, name or relative path=path "Anemometry/Anemometry Sub Vis/Gen Trav/Traverse_Space.vi") -> (appended path=w280:path)
            n223 = global read "Trav_pos_global.vi" "Default Traverse Setup"() -> (w272:string)
            n224 = Open VI Reference(type specifier VI Refnum (for type only)=refnum<vi> refnum, vi path=w280) -> (vi reference=w281:refnum<vi>, error out=w273:errorcluster)  [unwired: 1 in, 3 out]
            n225 = call-by-ref "?"(reference=w281, error in=w273, "Show Panel?"=w282, "Traverse Setup"=w272) -> (reference out=w275:refnum<vi>, error out=w274:errorcluster)  [unwired: 8 in, 1 out]
            n226 = Close Reference(reference=w275, error in (no error)=w274) -> ()  [unwired: 1 out]
            n227 = event-data("Discard?"=TRUE) -> ()  [unwired: 1 in, 4 out]
          }
          event Mouse Down? {
            n228 = event-data() -> ()  [unwired: 5 out]
            n229 = global read "Constants_global.vi" "EnFlo SW Folder"() -> (w284:path)
            n230 = Build Path(base path=w284, name or relative path=path "Anemometry/Anemometry Sub Vis/Traverse vi's/EnFlo Tunnel specific/Check_EnFlo_Arm.vi") -> (appended path=w286:path)
            n231 = call "Open_Close_Front_Panel.ph.vi"("Front Panel Window:Open"=TRUE, "VI path"=w286) -> ()  [unwired: 2 out]
            n232 = event-data() -> ()  [unwired: 1 in, 2 out]
          }
          event Mouse Down? {
            n233 = event-data() -> ()  [unwired: 5 out]
            n234 = global read "Constants_global.vi" "EnFlo SW Folder"() -> (w294:path)
            n235 = Build Path(base path=w294, name or relative path=path "Anemometry/Anemometry Sub Vis/Gen Trav/3D_Traverse_move.vi") -> (appended path=w291:path)
            n236 = Strip Path(path=w291) -> (name=w290:string)  [unwired: 1 out]
            n237 = Open VI Reference(vi path=w290) -> (vi reference=w292:refnum<vi>, error out=w293:errorcluster)  [unwired: 1 in, 4 out]
            n238 = property class="VI"(reference=w292, error in=w293) -> (reference out=w288:refnum<vi>, error out=w287:errorcluster, "Front Panel Window:Open"=w289:bool)
            n239 = case shown="False" w289 {
              tunnel: w291 -> [w296 _]
              tunnel: w288 -> [_ w313]
              tunnel: w287 -> [_ w312]
              frame False {
                n240 = global read "Trav_pos_global.vi" "Work in Tunnel Coordinates?"() -> (w306:T48)
                n241 = global read "Trav_pos_global.vi" "Default Traverse Setup"() -> (w304:string)
                n242 = Open VI Reference(type specifier VI Refnum (for type only)=refnum<vi> refnum, vi path=w296) -> (vi reference=w300:refnum<vi>, error out=w301:errorcluster)  [unwired: 1 in, 3 out]
                n243 = property class="VI Interface Type 4"(reference=w300, error in=w301, "Front Panel Window:Open"=TRUE) -> (reference out=w297:refnum<vi>, error out=w298:errorcluster)
                n244 = call-by-ref "?"(reference=w297, error in=w298, "Mode"=Trav_mode."Read traverse position", "Work in Tunnel Coordinates"=w306, "Simulate/Run"=User_Specific_mode."Run VI", "Traverse name"=w304) -> (reference out=w302:refnum<vi>, error out=w303:errorcluster)  [unwired: 9 in, 3 out]
                n245 = Close Reference(reference=w302, error in (no error)=w303) -> ()  [unwired: 1 out]
              }
              frame True {
                n246 = property class="VI"(reference=w313, error in=w312, "Front Panel Window:Open"=TRUE) -> (reference out=w311:refnum<vi>, error out=w310:errorcluster)
                n247 = Close Reference(reference=w311, error in (no error)=w310) -> ()  [unwired: 1 out]
              }
            }
            n248 = event-data() -> ()  [unwired: 1 in, 5 out]
          }
          event Mouse Down? {
            n249 = event-data() -> ()  [unwired: 5 out]
            n250 = Open VI Reference(vi path="Multi_Run_Prog.vi") -> (vi reference=w319:refnum<vi>, error out=w318:errorcluster)  [unwired: 1 in, 4 out]
            n251 = property class="VI"(reference=w319, error in=w318, "Front Panel Window:Open"=TRUE) -> (reference out=w316:refnum<vi>, error out=w317:errorcluster)
            n252 = Close Reference(reference=w316, error in (no error)=w317) -> (error out=w314:errorcluster)
            n253 = Unbundle By Name(w314) -> ("status"=w321:bool)
            n254 = case shown="True" w321 {
              frame False {
              }
              frame True {
                n255 = global read "Constants_global.vi" "EnFlo SW Folder"() -> (w329:path)
                n256 = call "Setup_Filepath.vi"("Setup File Type"=Setup_Filetype."General", "Filename in"="Multi_Run_Filename.txt" ("name or relative path")) -> ("Filename Out"=w322:path)  [unwired: 1 out]
                n257 = Build Path(base path=w329, name or relative path=path "Anemometry/Multi_Run_Prog.vi") -> (appended path=w328:path)
                n258 = call "Read_File_Simple.vi"("Filename"=w322) -> ("string"=w327:string)  [unwired: 2 in, 7 out]
                n259 = String To Path(string=w327) -> (path=w325:path)
                n260 = call "Does_file_exist_(simple).vi"("Pathname"=w325) -> ("exists?"=w326:bool)
                n261 = case shown="False" w326 {
                  tunnel: w328 -> [w331 w343]
                  tunnel: w325 -> [_ w340]
                  frame False {
                    n262 = call "Open_Close_Front_Panel.ph.vi"("Front Panel Window:Open"=TRUE, "VI path"=w331) -> ()  [unwired: 2 out]
                  }
                  frame True {
                    n263 = Open VI Reference(type specifier VI Refnum (for type only)=refnum<vi> refnum, vi path=w343) -> (vi reference=w339:refnum<vi>, error out=w338:errorcluster)  [unwired: 1 in, 3 out]
                    n264 = property class="VI Interface Type 5"(reference=w339, error in=w338, "Front Panel Window:Open"=TRUE) -> (reference out=w336:refnum<vi>, error out=w337:errorcluster)
                    n265 = call-by-ref "?"(reference=w336, error in=w337, "Command filename"=w340, "Setup mode"=T46."Load Command File") -> (reference out=w335:refnum<vi>, error out=w334:errorcluster)  [unwired: 18 in]
                    n266 = Close Reference(reference=w335, error in (no error)=w334) -> ()  [unwired: 1 out]
                  }
                }
              }
            }
            n267 = event-data() -> ()  [unwired: 1 in, 5 out]
          }
          event Mouse Down? {
            w345 = "Calibration.vi" ("name or relative path")
            n268 = event-data() -> ()  [unwired: 5 out]
            n269 = global read "Constants_global.vi" "EnFlo SW Folder"() -> (w351:path)
            n270 = Open VI Reference(vi path=w345) -> (vi reference=w349:refnum<vi>, error out=w348:errorcluster)  [unwired: 1 in, 4 out]
            n271 = Build Path(base path=w351, name or relative path="Anemometry") -> (appended path=w354:path)
            n272 = property class="VI"(reference=w349, error in=w348, "Front Panel Window:Open"=TRUE) -> (reference out=w346:refnum<vi>, error out=w347:errorcluster)
            n273 = Build Path(base path=w354, name or relative path=w345) -> (appended path=w352:path)
            n274 = Close Reference(reference=w346, error in (no error)=w347) -> (error out=w344:errorcluster)
            n275 = Unbundle By Name(w344) -> ("status"=w353:bool)
            n276 = case shown="True" w353 {
              tunnel: w352 -> [_ w356]
              tunnel: w344 -> [_ _]
              frame False {
              }
              frame True {
                n277 = stacked-sequence {
                  seq-local: [w362 _] -> [_ w369]
                  tunnel: w356 -> [_ w370]
                  frame #0 {
                    n278 = call "Setup_Filepath.vi"("Setup File Type"=Setup_Filetype."Calibration Setups", "Filename in"="Current_Setup.xls") -> ("Filename Out"=w357:path)  [unwired: 1 out]
                    n279 = call "Read_File_Simple.vi"("Filename"=w357) -> ("string"=w366:string)  [unwired: 2 in, 7 out]
                    n280 = Format Into String(format string="Calibration Setup File   %s", w357) -> (resulting string=w360:string)  [unwired: 2 in, 1 out]
                    n281 = call "Get_string_subset.vi"("String Name"=w360, "String to split"=w366, "File Label"="Raw data header") -> ("Output string"=w364:string)  [unwired: 1 in, 1 out]
                    n282 = call "Get_Characters_from_string.vi"("Input string"=w364, "Variable name"="Calib filename") -> ("Value"=w363:string)  [unwired: 1 in, 1 out]
                    n283 = call "String_to_Pathname.vi"("Input String"=w363) -> ("path"=w362:path)
                  }
                  frame #1 {
                    n284 = call "Does_file_exist_(simple).vi"("Pathname"=w369) -> ("exists?"=w368:bool)
                    n285 = case shown="True" w368 {
                      tunnel: w370 -> [w371 w386]
                      tunnel: w369 -> [_ w380]
                      frame False {
                        n286 = call "Open_Close_Front_Panel.ph.vi"("Front Panel Window:Open"=TRUE, "VI path"=w371) -> ()  [unwired: 2 out]
                      }
                      frame True {
                        w378 = TRUE ("Front Panel Window:Open")
                        n287 = Open VI Reference(type specifier VI Refnum (for type only)=refnum<vi> refnum, vi path=w386) -> (vi reference=w384:refnum<vi>, error out=w379:errorcluster)  [unwired: 1 in, 3 out]
                        n288 = property class="VI Interface Type 6"(reference=w384, error in=w379, "Front Panel Window:Open"=w378, "Front Panel Window:Auto Center (Deprecated)"=w378) -> (reference out=w383:refnum<vi>, error out=w382:errorcluster)
                        n289 = call-by-ref "?"(reference=w383, error in=w382, "Mode"=Calib_mode."Setup Front Panel", "Calib file"=w380) -> (reference out=w376:refnum<vi>, error out=w375:errorcluster)  [unwired: 15 in, 3 out]
                        n290 = property class="VI Interface Type 6"(reference=w376, error in=w375, "Front Panel Window:Auto Center (Deprecated)"=FALSE ("Front Panel Window:Auto Center")) -> (reference out=w374:refnum<vi>, error out=w373:errorcluster)
                        n291 = Close Reference(reference=w374, error in (no error)=w373) -> ()  [unwired: 1 out]
                      }
                    }
                  }
                }
              }
            }
            n292 = event-data() -> ()  [unwired: 1 in, 5 out]
          }
          event "stop": Mouse Down? {
            n293 = event-data() -> ()  [unwired: 5 out]
            n294 = flat-sequence {
              frame #0 {
                n295 = global write "Dynamic_call_global.ph.vi" "EnFlo Hub running?"(FALSE ("EnFlo Hub running?")) -> ()
              }
              frame #1 {
                n296 = Stop(stop? (T)=TRUE) -> ()
              }
            }
            n297 = event-data() -> ()  [unwired: 1 in, 4 out]
          }
          event "Rig_Control": Value Change {
            n298 = event-data() -> ("OldVal"=w390:cluster{"Ch Name":string, "Boolean":bool}[], "NewVal"=w389:cluster{"Ch Name":string, "Boolean":bool}[])  [unwired: 5 out]
            n299 = for {
              tunnel: w390 -> [w396] mode=indexing
              tunnel: w389 -> [w395] mode=indexing
              n300 = Unbundle By Name(w396) -> ("Ch Name"=w393:string, "Boolean"=w394:bool)
              n301 = Unbundle By Name(w395) -> ("Boolean"=w392:bool)  [unwired: 1 out]
              n302 = Not Equal?(x=w394, y=w392) -> (x != y?=w391:bool)
              n303 = case shown="True" w391 {
                tunnel: w393 -> [_ w398]
                tunnel: w392 -> [_ w405]
                frame False {
                }
                frame True {
                  n304 = Select(t="TRUE", s=w405, f="FALSE") -> (s? t:f=w397:string)
                  n305 = Select(t=1.0, s=w405, f=0.0) -> (s? t:f=w404:dbl)
                  n306 = Format Into String(format string="Are you sure you want to make %s %s?", w398, w397) -> (resulting string=w407:string)  [unwired: 2 in, 1 out]
                  n307 = Format Into String(format string="Make  %s  %s", w398, w397) -> (resulting string=w399:string)  [unwired: 2 in, 1 out]
                  n308 = Two Button Dialog(message=w407, 1:w399, 2:"Cancel" ("T button name (\"OK\")")) -> (T button?=w401:bool)
                  n309 = case shown="False" w401 {
                    tunnel: w398 -> [w412 _]
                    tunnel: w404 -> [w411 _]
                    frame False {
                      n310 = Build Array(w411) -> (w414:dbl[])
                      n311 = Build Array(w412) -> (w413:string[])
                      n312 = call "ASYNC_Adam_client.vi"("Values"=w414, "Channel Names"=w413) -> ()  [unwired: 2 out]
                    }
                    frame True {
                    }
                  }
                }
              }
            }
          }
          event Mouse Down? {
            w421 = TRUE  # Show Panel
            w420 = path "Anemometry/Anemometry Sub Vis/LDA/Enter_LDA_Setup.vi"  # :Anemometry:Anemometry Sub Vis:LDA:Enter_LDA_Setup.vi
            n313 = event-data() -> ()  [unwired: 5 out]
            n314 = global read "Constants_global.vi" "EnFlo SW Folder"() -> (w415:path)
            n315 = Build Path(base path=w415, name or relative path=w420) -> (appended path=w419:path)
            n316 = Open VI Reference(type specifier VI Refnum (for type only)=refnum<vi> refnum, vi path=w419) -> (vi reference=w422:refnum<vi>, error out=w423:errorcluster)  [unwired: 1 in, 3 out]
            n317 = call-by-ref "?"(reference=w422, error in=w423, "Show Panel"=w421) -> (reference out=w417:refnum<vi>, error out=w418:errorcluster)
            n318 = Close Reference(reference=w417, error in (no error)=w418) -> ()  [unwired: 1 out]
            n319 = event-data() -> ()  [unwired: 1 in, 4 out]
          }
        }
      }
    }
    "Numeric" <- w8
  }
  n320 = while {
    shift-left: _ -> [w428]
    shift-right: [w429] -> _
    shift-left: "Initialise" -> [w427]
    shift-right: [w430] -> _
    tunnel: "ADAM_Chs_to_Enable.txt" ("name or relative path") -> [w425]
    tunnel: "ADAM_Chs_to_View.txt" ("name or relative path") -> [w424]
    i -> [w426]
    stop <- TRUE continue-if-true
    n321 = case shown="\"Initialise\"" w427 {
      tunnel: ["End" "Initialise" "Wait for call remote sub vi occurrence" "Check type of VI to launch" w503 "Wait until remote sub vi is opened" "Update opened vis array" "Update opened vis array" "Update opened vis array" "Wait until remote sub vi is opened" "Wait for call remote sub vi occurrence"] -> w430
      tunnel: [w432 w447 w452 errorcluster {"status"=FALSE, "code"=0, "source"=""} ("error out") w499 w514 w544 w561 w576 w616 w636] -> w429
      tunnel: w428 -> [w432 w447 w452 _ w499 w514 _ _ _ w616 w636]
      tunnel: w427 -> [w434 _ _ _ _ _ _ _ _ _ _]
      tunnel: w426 -> [_ _ _ _ _ _ _ _ _ _ _]
      tunnel: w425 -> [_ _ w449 _ _ _ _ _ _ _ _]
      tunnel: w424 -> [_ _ w448 _ _ _ _ _ _ _ _]
      frame "No match", Default {
        n322 = Current VI's Path() -> (path=w435:path)
        n323 = Format Into String(format string="The Case\"%s\" was not Matched\nin VI named\n'%s\"" ("Format String"), w434, w435) -> (resulting string=w438:string)  [unwired: 2 in, 1 out]
        n324 = One Button Dialog(message=w438, button name ("OK")="STOP") -> (true=w436:bool)
        n325 = Stop(stop? (T)=w436) -> ()
      }
      frame "Never run" {
        # "These globals are here to make sure they stay in momory\nafter \"Preference Panel\" has finished running"
        n326 = call "Email_With_Log.vi"() -> ()  [unwired: 4 in, 3 out]
        n327 = call "Remember_value.vi"() -> ()  [unwired: 3 in, 1 out]
        n328 = call "Read_Write_Local_table.vi"() -> ()  [unwired: 3 in, 3 out]
        n329 = call "Overhead_Factor.vi"() -> ()  [unwired: 4 in, 1 out]
        n330 = global read "Trav_pos_global.vi" "Dummy Measurement?"() -> (→"Dummy Measurement":bool)
        n331 = global read "PWAtasksGLOBAL.vi" "Analogue Dev Name"() -> (→"Analogue Dev Name":string)
        n332 = global read "Dynamic_call_global.ph.vi" "Ready to take data?"() -> (→"Ready to take data?":T1)
        n333 = global read "Qnet_Globals.vi" "Local Site Root"() -> (→"Local Site Root":path)
        n334 = global read "Constants_global.vi" "All_Users"() -> (→"All Users":path)
        n335 = global read "Preference_global.vi" "Rig Setup"() -> (→"Rig Name":string)
      }
      frame "Initialise" {
        n336 = stacked-sequence {
          tunnel: w449 -> [_ _ _ _ w491]
          tunnel: w448 -> [_ _ _ _ w487]
          frame #0 {
            n337 = Generate Occurrence() -> (w474:refnum<k4>)
            n338 = global write "Dynamic_call_global.ph.vi" "Call Remote Subvi"(w474) -> ()
            n339 = Generate Occurrence() -> (w473:refnum<k4>)
            n340 = global write "Dynamic_call_global.ph.vi" "Remote Subvi Opened"(w473) -> ()
            n341 = Initialize Array("", 0) -> (w471:string[])
            n342 = global write "Dynamic_call_global.ph.vi" "Opened VIs"(w471) -> ()
            n343 = global write "Email_transfer_global.vi" "Busy?"(FALSE ("Busy?")) -> ()
            n344 = Current VI's Path() -> (path=w463:path)
            n345 = Strip Path(path=w463) -> (stripped path=w461:path)  [unwired: 1 out]
            n346 = Build Path(base path=w461, name or relative path="Utilities") -> (appended path=w459:path)
            n347 = Build Path(base path=w459, name or relative path="Preference_Panel.vi") -> (appended path=w458:path)
            n348 = Get Date/Time In Seconds() -> (seconds since 1Jan1904=w469:timestamp)
            n349 = To Double Precision Float(number=w469) -> (double precision float=w468:dbl)
            n350 = Open VI Reference(type specifier VI Refnum (for type only)=refnum<vi> refnum, vi path=w458) -> (vi reference=w464:refnum<vi>, error out=w465:errorcluster)  [unwired: 1 in, 3 out]
            n351 = Generate Occurrence() -> (w454:refnum<k4>)
            n352 = global write "Meas_global.vi" "Start Time of experiment"(w468) -> ()
            n353 = global write "Meas_global.vi" "Post Process"(Post_Process."Post Process Raw Data File" ("Post Process")) -> ()
            n354 = call-by-ref "?"(reference=w464, error in=w465, "Mode"=Preference_Mode."Load Preferences from file") -> (reference out=w466:refnum<vi>, error out=w467:errorcluster)
            n355 = global write "Dynamic_call_global.ph.vi" "Take data"(w454) -> ()
            n356 = Close Reference(reference=w466, error in (no error)=w467) -> ()  [unwired: 1 out]
          }
          frame #1 {
            w475 = TRUE  # OK
            n357 = call "Get_users_email_addresses.vi"("OK"=w475) -> ()  [unwired: 5 out]
          }
          frame #2 {
            n358 = Current VI's Path() -> (path=w484:path)
            n359 = Open VI Reference(vi path=w484) -> (vi reference=w483:refnum<vi>, error out=w482:errorcluster)  [unwired: 1 in, 4 out]
            n360 = call "Last_modified_date.vi"("Update Now"=TRUE) -> ("Programs last revision time"=w477:u32)  [unwired: 1 out]
            n361 = property class="VI"(reference=w483, error in=w482, "Front Panel Window:Open"=TRUE, "Front Panel Window:Is Frontmost"=FALSE) -> (reference out=w481:refnum<vi>, error out=w480:errorcluster)
            n362 = global write "Meas_global.vi" "Prog's last revision date"(w477) -> ()
            n363 = Close Reference(reference=w481, error in (no error)=w480) -> ()  [unwired: 1 out]
          }
          frame #3 {
            n364 = global write "Dynamic_call_global.ph.vi" "EnFlo Hub running?"(TRUE ("EnFlo Hub running?")) -> ()
          }
          frame #4 {
            n365 = global read "Constants_global.vi" "All_Users"() -> (w488:path)
            n366 = Build Path(base path=w488, name or relative path=w487) -> (appended path=w490:path)
            n367 = Build Path(base path=w488, name or relative path=w491) -> (appended path=w493:path)
            n368 = call "Read_File_Simple.vi"("Filename"=w490) -> ("string"=w489:string)  [unwired: 2 in, 7 out]
            n369 = call "Read_File_Simple.vi"("Filename"=w493) -> ("string"=w494:string)  [unwired: 2 in, 7 out]
            n370 = call "Get_array_values_fr_String.vi"("String Value"=w489) -> ("String array"=→"List of ADAM channels to view":string[])  [unwired: 1 out]
            n371 = call "Get_array_values_fr_String.vi"("String Value"=w494) -> ("String array"=→"List of ADAM control channels":string[])  [unwired: 1 out]
          }
        }
        "Iterations" <- 0 ("Iterations")
      }
      frame "Wait for call remote sub vi occurrence" {
        n372 = global read "Dynamic_call_global.ph.vi" "Call Remote Subvi"() -> (w497:refnum<k4>)
        n373 = Wait on Occurrence(2:w497) -> ()  [unwired: 3 out]
      }
      frame "Check type of VI to launch" {
        n374 = global read "Dynamic_call_global.ph.vi" "VI name to launch"() -> (w501:string)
        n375 = Match Pattern(string=w501, regular expression=";") -> (before substring=w498:string, after substring=w500:string)  [unwired: 3 out]
        n376 = case shown="\"Open LDA PWA & An\"" w498 {
          tunnel: ["Open vi" "Open application reference" "Open Analogue input server" w511] -> w503
          tunnel: [w506 w508 w510 w512] -> w502
          tunnel: w501 -> [w506 _ _ _]
          tunnel: w500 -> [_ w508 w510 w512]
          tunnel: w498 -> [_ _ _ w511]
          frame "Other", Default {
          }
          frame "Open Application Reference" {
          }
          frame "Open Analogue Input VI" {
          }
          frame "Open LDA PWA & An" {
          }
        }
        "VI Name" <- w502
      }
      frame "Open application reference" {
        n377 = local read "VI Name"() -> (w515:string)
        n378 = Match Pattern(string=w515, regular expression=";") -> (before substring=w523:string, after substring=w524:string)  [unwired: 3 out]
        n379 = Decimal String To Number(string=w524) -> (number=w525:i32)  [unwired: 3 out]
        n380 = To Unsigned Long Integer(number=w525) -> (unsigned 32bit integer=w522:u32)
        n381 = call "App_Ref_Global.vi"("Mode"=App_Global."Read Global") -> ("Output Array"=w521:T50[])  [unwired: 1 in, 1 out]
        n382 = Open Application Reference(10:w522, 11:w523) -> (0:w516:errorcluster, 3:w520:refnum<vi>)  [unwired: 1 in, 1 out]
        n383 = for {
          tunnel: w521 -> [w527] mode=indexing
          tunnel: w515 -> [w531]
          tunnel: w520 -> [w529]
          tunnel: [w528] -> w519 mode=indexing
          n384 = Unbundle By Name(w527) -> ("Server IP & Port No"=w532:string)
          n385 = Equal?(x=w532, y=w531) -> (x = y?=w530:bool)
          n386 = case shown="False" w530 {
            tunnel: w529 -> [_ w536]
            tunnel: [w533 w535] -> w528
            tunnel: w527 -> [w533 w534]
            frame False {
            }
            frame True {
              n387 = Bundle By Name(cluster=w534, "Application reference"=w536) -> (w535:T50)
            }
          }
        }
        n388 = global write "Dynamic_call_global.ph.vi" "Error Cluster"(w516) -> ()
        n389 = call "App_Ref_Global.vi"("Input Array"=w519, "Mode"=App_Global."Write to Global") -> ()  [unwired: 2 out]
      }
      frame "Open Analogue input server" {
        n390 = local read "VI Name"() -> (w541:string)
        n391 = call "Get_link_info.vi"("VI Name"=w541) -> ("Path name"=w538:path, "Application reference"=w539:refnum<vi>, "Local Call?"=w540:bool)  [unwired: 1 out]
        n392 = global read "Dynamic_call_global.ph.vi" "Analogue Input"() -> (w543:refnum<vi>)
        n393 = case shown="True" w540 {
          tunnel: w543 -> [w549 w553]
          tunnel: [w545 w552] -> w542
          tunnel: [w548 w551] -> w544
          tunnel: w541 -> [w547 _]
          tunnel: w539 -> [w546 _]
          tunnel: w538 -> [_ w550]
          frame False {
            n394 = Open VI Reference(type specifier VI Refnum (for type only)=w549, application reference (local)=w546, vi path=w547) -> (vi reference=w545:refnum<vi>, error out=w548:errorcluster)  [unwired: 1 in, 2 out]
          }
          frame True {
            n395 = Open VI Reference(type specifier VI Refnum (for type only)=w553, vi path=w550) -> (vi reference=w552:refnum<vi>, error out=w551:errorcluster)  [unwired: 1 in, 3 out]
          }
        }
        n396 = global write "Dynamic_call_global.ph.vi" "Analogue Input"(w542) -> ()
      }
      frame "Open LDA PWA & An" {
        n397 = local read "VI Name"() -> (w558:string)
        n398 = call "Get_link_info.vi"("VI Name"=w558) -> ("Path name"=w555:path, "Application reference"=w556:refnum<vi>, "Local Call?"=w557:bool)  [unwired: 1 out]
        n399 = global read "Dynamic_call_global.ph.vi" "Take LDA PWA & An"() -> (w560:refnum<vi>)
        n400 = case shown="True" w557 {
          tunnel: w560 -> [w566 w570]
          tunnel: [w562 w569] -> w559
          tunnel: [w565 w568] -> w561
          tunnel: w558 -> [w564 _]
          tunnel: w556 -> [w563 _]
          tunnel: w555 -> [_ w567]
          frame False {
            n401 = Open VI Reference(type specifier VI Refnum (for type only)=w566, application reference (local)=w563, vi path=w564) -> (vi reference=w562:refnum<vi>, error out=w565:errorcluster)  [unwired: 1 in, 2 out]
          }
          frame True {
            n402 = Open VI Reference(type specifier VI Refnum (for type only)=w570, vi path=w567) -> (vi reference=w569:refnum<vi>, error out=w568:errorcluster)  [unwired: 1 in, 3 out]
          }
        }
        n403 = global write "Dynamic_call_global.ph.vi" "Take LDA PWA & An"(w559) -> ()
      }
      frame "Open vi" {
        n404 = local read "VI Name"() -> (w575:string)
        n405 = call "Get_link_info.vi"("VI Name"=w575) -> ("Path name"=w574:path, "Application reference"=w573:refnum<vi>, "Local Call?"=w572:bool)  [unwired: 1 out]
        n406 = case shown="\"No Match\", Default" w575 {
          tunnel: [w577 w586 w598] -> w576
          tunnel: w575 -> [w582 w585 w602]
          tunnel: w574 -> [_ _ w599]
          tunnel: w573 -> [_ w584 w601]
          tunnel: w572 -> [_ w583 w600]
          frame "No Match", Default {
            n407 = Format Into String(format string="VI named \"%s\" Not matched" ("Format String"), w582) -> (resulting string=w579:string)  [unwired: 2 in, 1 out]
            n408 = Bundle By Name(cluster=errorcluster {"status"=FALSE, "code"=0, "source"=""} ("error out"), "source"=w579, "status"=TRUE ("Bundle Element")) -> (w577:errorcluster)
          }
          frame "Program_Active_server.vi" {
            n409 = global read "Dynamic_call_global.ph.vi" "Program Active server"() -> (w588:refnum<vi>)
            n410 = case shown="True" w583 {
              tunnel: w588 -> [w593 w597]
              tunnel: [w592 w596] -> w587
              tunnel: [w591 w595] -> w586
              tunnel: w585 -> [w590 w594]
              tunnel: w584 -> [w589 _]
              frame False {
                n411 = Open VI Reference(type specifier VI Refnum (for type only)=w593, application reference (local)=w589, vi path=w590) -> (vi reference=w592:refnum<vi>, error out=w591:errorcluster)  [unwired: 1 in, 2 out]
              }
              frame True {
                n412 = Open VI Reference(type specifier VI Refnum (for type only)=w597, vi path=w594) -> (vi reference=w596:refnum<vi>, error out=w595:errorcluster)  [unwired: 1 in, 3 out]
              }
            }
            n413 = global write "Dynamic_call_global.ph.vi" "Program Active server"(w587) -> ()
          }
          frame "GPIB_Server.vi" {
            n414 = global read "Dynamic_call_global.ph.vi" "GPIB_Server.vi"() -> (w604:refnum<vi>)
            n415 = case shown="False" w600 {
              tunnel: w604 -> [w609 w613]
              tunnel: [w608 w612] -> w603
              tunnel: [w607 w611] -> w598
              tunnel: w602 -> [w605 _]
              tunnel: w601 -> [w606 _]
              tunnel: w599 -> [_ w610]
              frame False {
                n416 = Open VI Reference(type specifier VI Refnum (for type only)=w609, application reference (local)=w606, vi path=w605) -> (vi reference=w608:refnum<vi>, error out=w607:errorcluster)  [unwired: 1 in, 2 out]
              }
              frame True {
                n417 = Open VI Reference(type specifier VI Refnum (for type only)=w613, vi path=w610) -> (vi reference=w612:refnum<vi>, error out=w611:errorcluster)  [unwired: 1 in, 3 out]
              }
            }
            n418 = global write "Dynamic_call_global.ph.vi" "GPIB_Server.vi"(w603) -> ()
          }
        }
      }
      frame "Update opened vis array" {
        w618 = TRUE  # Dialog Box
        n419 = local read "VI Name"() -> (w617:string)
        n420 = Unbundle By Name(w616) -> ("status"=w621:bool, "source"=w619:string)
        n421 = case shown="True" w621 {
          tunnel: w616 -> [w623 w632]
          tunnel: [w623 w631] -> w620
          tunnel: w617 -> [w624 w627]
          tunnel: w619 -> [_ w630]
          frame False {
            n422 = global read "Dynamic_call_global.ph.vi" "Opened VIs"() -> (w625:string[])
            n423 = To Upper Case(1:w624) -> (0:w622:string)
            n424 = Build Array (concatenate)(w625, w622) -> (w626:string[])
            n425 = global write "Dynamic_call_global.ph.vi" "Opened VIs"(w626) -> ()
          }
          frame True {
            n426 = Concatenate Strings(w627, " " ("Substring"), w630) -> (w628:string)
            n427 = Bundle By Name(cluster=w632, "source"=w628) -> (w631:errorcluster)
          }
        }
        n428 = call "EnFlo_Error_Handler.vi"("error in (no error)"=w620, "Error Type"="Dynamic Call", "Dialog Box (T)"=w618) -> ()  [unwired: 3 out]
      }
      frame "Wait until remote sub vi is opened" {
        n429 = global read "Dynamic_call_global.ph.vi" "Remote Subvi Opened"() -> (w637:refnum<k4>)
        n430 = local read "Iterations"() -> (w635:i32)
        n431 = Increment(x=w635) -> (x+1=w634:i32)
        n432 = local write "Iterations"(w634) -> ()
        n433 = Set Occurrence(w637) -> ()
      }
    }
  }
  n434 = while {
    stop <- FALSE stop-if-true
    n435 = global read "Dynamic_call_global.ph.vi" "EnFlo Hub running?"() -> (w639:bool)
    n436 = Equal?(x="Tab Control", y=T2."Adam Table" ("Tab Control")) -> (x = y?=w640:bool)
    n437 = And(x=w640, y=w639) -> (x .and. y?=w638:bool)
    n438 = case shown="True" w638 {
      frame True {
        n439 = local read "List of ADAM channels to view"() -> (w651:string[])
        n440 = local read "List of ADAM control channels"() -> (w654:string[])
        n441 = Build Array (concatenate)(w654, w651) -> (w653:string[])
        n442 = call "Get_Current_Scan_client.vi"("ADAM Ch Names"=w653) -> ("Ch Description Array"=w648:T51[], "Numerical Values"=w652:dbl[])  [unwired: 2 out]
        n443 = Array Size(array=w654) -> (size(s)=w649:i32)
        n444 = Array Subset(array=w648, index=w649) -> (w647:T51[])  [unwired: 1 in]
        n445 = Array Subset(array=w652, index=w649) -> (w646:dbl[])  [unwired: 1 in]
        n446 = for {
          tunnel: w647 -> [w661] mode=indexing
          tunnel: [w660] -> w645 mode=indexing
          tunnel: cluster{"Ch Name":string, "Numeric":dbl} {"Ch Name"="", "Numeric"=0.0} ("Cluster") -> [w659]
          tunnel: w646 -> [w657] mode=indexing
          n447 = Unbundle By Name(w661) -> ("Ch Name"=w658:string)
          n448 = Bundle By Name(cluster=w659, "Ch Name"=w658, "Numeric"=w657) -> (w660:cluster{"Ch Name":string, "Numeric":dbl})
        }
        "Current Values" <- w645
        n449 = for {
          N: w649 -> [_]
          tunnel: cluster{"Ch Name":string, "Boolean":bool} {"Ch Name"="", "Boolean"=FALSE} ("Cluster") -> [w668]
          tunnel: w648 -> [w667] mode=indexing
          tunnel: w652 -> [w665] mode=indexing
          tunnel: [w662] -> w655 mode=indexing
          n450 = Unbundle By Name(w667) -> ("Ch Name"=w666:string)
          n451 = Greater?(x=w665, y=0.5) -> (0:w663:bool)
          n452 = Bundle By Name(cluster=w668, "Ch Name"=w666, "Boolean"=w663) -> (w662:cluster{"Ch Name":string, "Boolean":bool})
        }
        n453 = local write "Rig_Control"(w655) -> ()
      }
      frame False {
      }
    }
    n454 = Wait (ms)(milliseconds to wait=u32 1000) -> ()  [unwired: 1 out]
  }
